vi "All Tubes ON - OFF.vi"(6 "Tubes ON/OFF":bool) -> ()   [LabVIEW 2020]
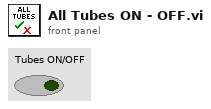
[diagram p1: front panel]
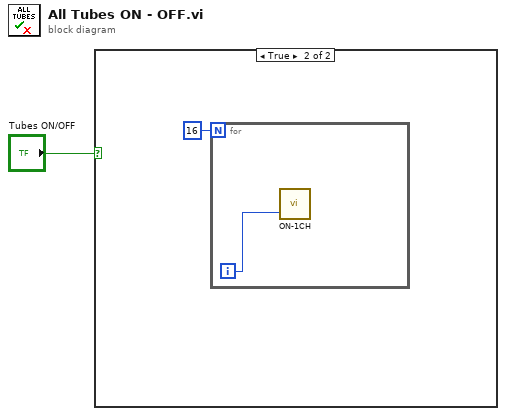
[diagram p0: block diagram]
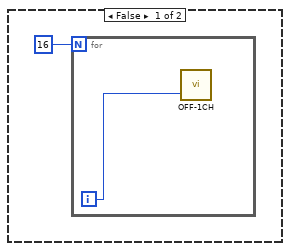
[diagram p2: hidden frame]
diagram:
  n1 = case shown="True" "Tubes ON/OFF" {
    frame False {
      n2 = for {
        N: 16 -> [_]
        i -> [w3]
        n3 = call "OFF-1CH.vi"("CH(0-63)"=w3) -> ()  [unwired: 1 in, 1 out]
      }
    }
    frame True {
      n4 = for {
        N: 16 -> [_]
        i -> [w5]
        n5 = call "ON-1CH.vi"("CH(0-63)"=w5) -> ()  [unwired: 1 in, 1 out]
      }
    }
  }
